vi "Test Sim data.vi"() -> ()   [LabVIEW 2013]
panel:
  out "sim data":u64[](array[numeric])
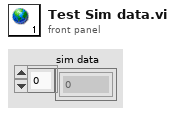
[diagram p1: front panel]
diagram:
